vi "Get Motors Position.vi"(8 "error in (no error)":errorcluster, 11 "KUKA youBot arm in":refnum<class "NI_Robotics_KUKA youBot Arm.lvclass">) -> (0 "error out":errorcluster, 2 "ccw position (rad)":dbl[](array[numeric]), 3 "KUKA youBot arm out":refnum<class "NI_Robotics_KUKA youBot Arm.lvclass">)   [LabVIEW 2017, in "NI_Robotics_KUKA youBot Host.lvlib" / "NI_Robotics_KUKA youBot Arm.lvclass"]
doc: "Gets the motors position, which the position encoder senses, of the joints of a KUKA youBot arm."
uses:
  <vilib>/robotics/KUKA youBot/Basic Device/Arm/NI_Robotics_KUKA youBot Arm.lvclass
  <vilib>/robotics/KUKA youBot/Basic Device/Arm/NI_Robotics_KUKA youBot Arm.lvclass/NI_Robotics_KUKA youBot Arm.ctl
  <vilib>/robotics/KUKA youBot/Motor/Arm Motor/NI_Robotics_KUKA youBot Arm Motor.lvclass
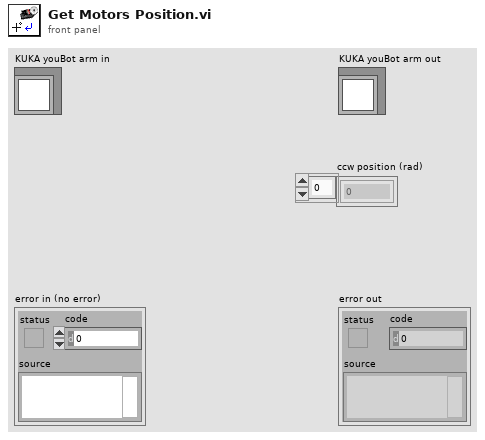
[diagram p1: front panel]
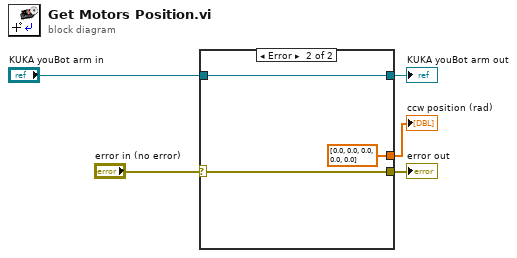
[diagram p0: block diagram]
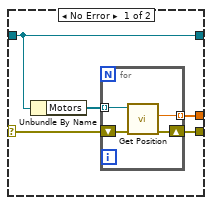
[diagram p2: hidden frame]
diagram:
  n1 = case shown="Error" "error in (no error)" {
    selector: "error in (no error)" -> [w6 w16]
    tunnel: [w7 w16] -> w1
    tunnel: [w10 w17] -> w3
    tunnel: "KUKA youBot arm in" -> [w10 w17]
    tunnel: [w8 dbl[] [0.0, 0.0, 0.0, 0.0, 0.0]] -> w2
    frame No Error {
      n2 = Unbundle By Name(w10) -> ("Motors"=w9:refnum<class "NI_Robotics_KUKA youBot Arm Motor.lvclass">[])
      n3 = for {
        tunnel: w9 -> [w14] mode=indexing
        tunnel: [w13] -> w8 mode=indexing
        shift-right: [w12] -> w7
        shift-left: w6 -> [w11]
        n4 = call-dynamic "Get Position.vi"("error in (no error)"=w11, "KUKA youBot arm motor in"=w14) -> ("error out"=w12:errorcluster, "CCW position (rad)"=w13:dbl)  [unwired: 7 in, 1 out]
      }
    }
    frame Error {
    }
  }
  "error out" <- w1
  "KUKA youBot arm out" <- w3
  "ccw position (rad)" <- w2
